vi "Stop Core.vi"(10 "final error code":i32, 11 "Example Controller Actor In":refnum<class "Example Controller.lvclass">) -> (3 "Example Controller Actor Out":refnum<class "Example Controller.lvclass">)   [LabVIEW 2023, in "Example GUI View.lvlib" / "Example Controller.lvclass"]
doc: "(<B>Filename</B>: Actor Framework.lvlib:Actor.lvclass:Stop Core.vi)\n\nDefines what the actor does before it stops. Use the <B>final error code</B> input to determine whether the actor shut down in response to an error.\n\nBy default, this method does nothing. A descendant class may override it to define behavior, such as shutting down any processes the actor initiated in its override of the Actor Core method."
uses:
  Example Controller.lvclass
  Example Controller.lvclass/Example Controller.ctl
  Example Controller/Example Controller/Example Controller.lvclass
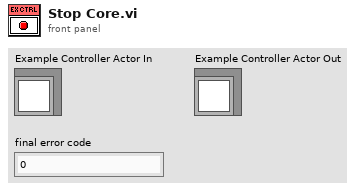
[diagram p1: front panel]
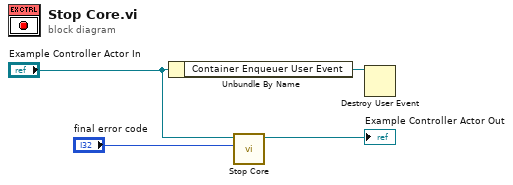
[diagram p0: block diagram]
diagram:
  n1 = Unbundle By Name("Example Controller Actor In") -> ("Container Enqueuer User Event"=w1:refnum<user-event>)
  n2 = call-parent "Stop Core.vi"("final error code"="final error code", "Controller In"="Example Controller Actor In") -> ("Controller Out"=→"Example Controller Actor Out":refnum<class "Example Controller.lvclass">)  [unwired: 9 in]
  n3 = Destroy User Event(user event=w1) -> ()  [unwired: 1 in, 1 out]
